vi "UpdateCurrentPosition.vi"(8 "error in (no error)":errorcluster, 11 "KST101 in":refnum<class "KST101.lvclass">) -> (0 "error out":errorcluster, 3 "KST101 out":refnum<class "KST101.lvclass">)   [LabVIEW 2016, in "Stepper Motor Controller.lvlib" / "KST101.lvclass"]
uses:
  KST101.lvclass
  KST101.lvclass/KST101.ctl
  D:/Workspace/ProCyteOne_LaserModuleAlignment/shared/Thorlabs/Kinesis/Dependencies/Thorlabs.MotionControl.KCube.StepperMotorCLI.dll
  Dependencies/Thorlabs.MotionControl.KCube.StepperMotorCLI.dll
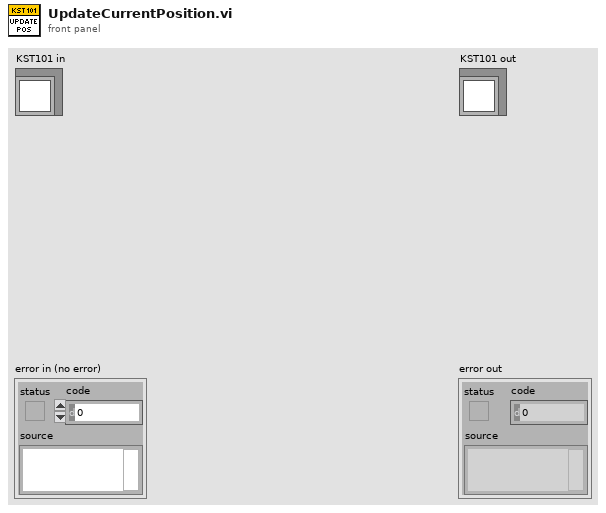
[diagram p1: front panel]
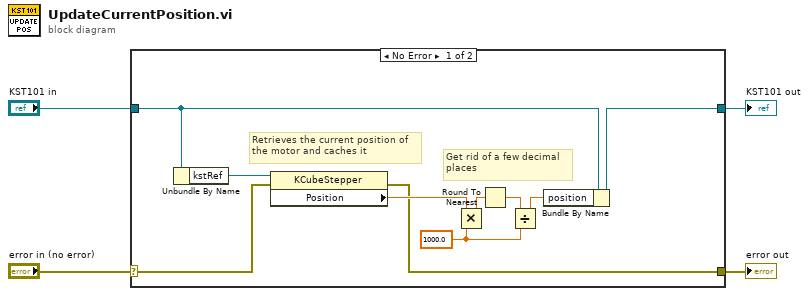
[diagram p0: block diagram]
diagram:
  n1 = case shown="No Error" "error in (no error)" {
    selector: "error in (no error)" -> [w10 w16]
    tunnel: [w9 w16] -> w3
    tunnel: [w13 w15] -> w1
    tunnel: "KST101 in" -> [w14 w15]
    frame No Error {
      w5 = 1000.0 ("y")
      # "Get rid of a few decimal\nplaces"
      # "Retrieves the current position of\nthe motor and caches it"
      n2 = Unbundle By Name(w14) -> ("kstRef"=w12:refnum<k24>)
      n3 = property class="KCubeStepper"(reference=w12, error in=w10) -> (error out=w9:errorcluster, "Position"=w11:dbl)  [unwired: 1 out]
      n4 = Multiply(x=w11, y=w5) -> (x*y=w8:dbl)
      n5 = Round To Nearest(number=w8) -> (nearest integer value=w7:dbl)
      n6 = Divide(x=w7, y=w5) -> (x/y=w6:dbl)
      n7 = Bundle By Name(cluster=w14, "position"=w6) -> (w13:refnum<class "KST101.lvclass">)
    }
    frame Error {
    }
  }
  "error out" <- w3
  "KST101 out" <- w1
